vi "Validate Custom Device Order.vi"(8 "error in (no error)":errorcluster, 11 "Device Item Ref in":T1 format="%.0x") -> (0 "error out":errorcluster, 3 "Device Item Ref out":T1 format="%.0x")   [LabVIEW 2020, in "Routing and Faulting System Explorer.lvlib"]
uses:
  Routing and Faulting System Explorer.lvlib
  <vilib>/NI VeriStand/Custom Device API/Custom Device Item Ref.ctl
  <vilib>/NI VeriStand/Custom Device API/Custom Device API.lvlib
  Shared/Routing and Faulting Hardware API/Routing and Faulting Hardware API.lvlib
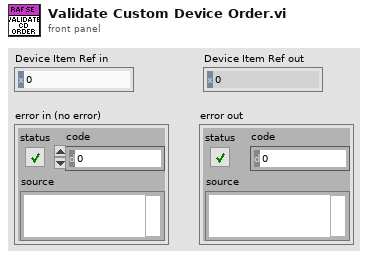
[diagram p1: front panel]
types:
  T1 = typedef "Custom Device API.lvlib/Custom Device Item Ref.ctl" = u64
  T2 = typedef "Custom Device API.lvlib/Custom Device Item Info.ctl" = cluster{"Name":string, "Is Channel":bool, "GUID":string, "Is Waveform":bool}
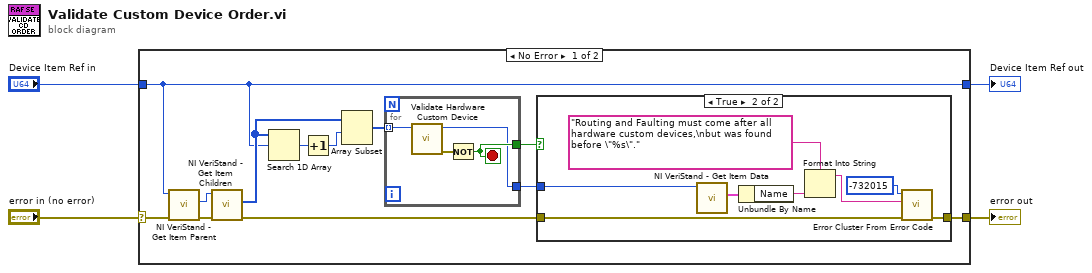
[diagram p0: block diagram]
diagram:
  n1 = case shown="No Error" "error in (no error)" {
    selector: "error in (no error)" -> [w10 w31]
    tunnel: [w15 w31] -> w4
    tunnel: "Device Item Ref in" -> [w6 w30]
    tunnel: [w6 w30] -> w1
    frame No Error {
      n2 = call <vilib>:"NI VeriStand - Get Item Parent.vi"("error in (no error)"=w10, "Item Ref in"=w6) -> ("error out"=w8:errorcluster, "Parent Ref"=w9:T1)  [unwired: 6 in, 2 out]
      n3 = call <vilib>:"NI VeriStand - Get Item Children.vi"("error in (no error)"=w8, "Item Ref in"=w9) -> ("error out"=w16:errorcluster, "Child Refs"=w7:T1[])  [unwired: 6 in, 2 out]
      n4 = Search 1D Array(1D array=w7, element=w6) -> (index of element=w11:i32)  [unwired: 1 in]
      n5 = Increment(x=w11) -> (x+1=w12:i32)
      n6 = Array Subset(array=w7, index=w12) -> (w5:T1[])  [unwired: 1 in]
      n7 = for {
        tunnel: w5 -> [w29] mode=indexing
        tunnel: [w27] -> w13
        tunnel: [w26] -> w14
        stop <- w27 stop-if-true
        n8 = call "Validate Hardware Custom Device.vi"("Hardware Ref in"=w29) -> ("error out"=w28:errorcluster, "Hardware Ref out"=w26:T1)  [unwired: 9 in]
        n9 = Not(x=w28) -> (.not. x?=w27:bool)
      }
      n10 = case shown="True" w13 {
        tunnel: w14 -> [_ w25]
        tunnel: [w17 w20] -> w15
        tunnel: w16 -> [w17 w19]
        frame False {
        }
        frame True {
          n11 = call <vilib>:"NI VeriStand - Get Item Data.vi"("Item Ref in"=w25) -> ("Item Info"=w24:T2)  [unwired: 7 in, 3 out]
          n12 = Unbundle By Name(w24) -> ("Name"=w23:string)
          n13 = Format Into String(format string="Routing and Faulting must come after all hardware custom devices,\nbut was found before \"%s\".", w23) -> (resulting string=w21:string)  [unwired: 2 in, 1 out]
          n14 = call <vilib>:"Error Cluster From Error Code.vi"("error in (no error)"=w19, "error message (\"\")"=w21, "error code (0)"=-732015) -> ("error out"=w20:errorcluster)  [unwired: 6 in]
        }
      }
    }
    frame Error {
    }
  }
  "error out" <- w4
  "Device Item Ref out" <- w1
